vi "onProcessKill.vi"(11 "SMO in":refnum<class "SMO.lvclass">) -> (3 "SMO out":refnum<class "SMO.lvclass">)   [LabVIEW 2019, in "SMO.lvclass"]
doc: "JKI State Machine Objects (SMO) 1.3.0.56\nJKI - JKI\nCopyright (c) 2017, JKI"
uses:
  SMO.lvclass
panel:
  # "This method is called if the call chain of the SMO\nis leaving memory while the process is running.\nAssume all references created in caller's thread to\nbe invalid."
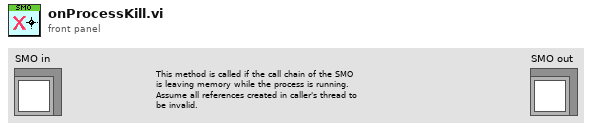
[diagram p1: front panel]
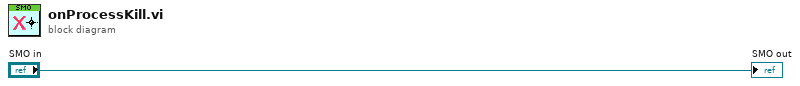
[diagram p0: block diagram]
diagram:
  "SMO out" <- "SMO in"
